vi "x1_move1.vi"() -> (0 "Enum":T1(ring))   [LabVIEW 2016]
uses:
  <vilib>/NXT/Block Support/NXT_OutputPort.ctl
  <vilib>/NXT/NXTIO Xnodes/NXTIONodeSubVIs/NXTMotorRunDistance.vi
  <vilib>/NXT/NXTIO Xnodes/NXTIONodeSubVIs/NXTMoveMotors.vi
  <vilib>/NXT/NXTIO Xnodes/NXTIONodeSubVIs/LEGOMotorStatus.vi
  <vilib>/NXT/NXTIO Xnodes/NXTIONodeSubVIs/NXTStopMotors.vi
  <vilib>/NXT/NXTIO Xnodes/NXTIONodeSubVIs/LEGOResetMotors.vi
  <vilib>/NXT/NXTIO Xnodes/AddressXNode/NXTIOAddress.xnode
  <vilib>/NXT/Subs/LVHSConnector.ctl
  <vilib>/NXT/NXTIO Xnodes/NXTIOXNode/NXTIO.xnode
  <vilib>/NXT/LegoClasses/BrickReference/BrickReference.lvclass
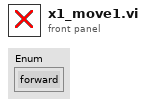
[diagram p1: front panel]
types:
  T1 = enum16{"forward", "mark", "pause", "up", "return", "end"}
  T2 = typedef "NXT_OutputPort.ctl" = u8
  T3 = cluster{"Output Port":T2, "Output Port 2":T2, "Output Port 3":T2}
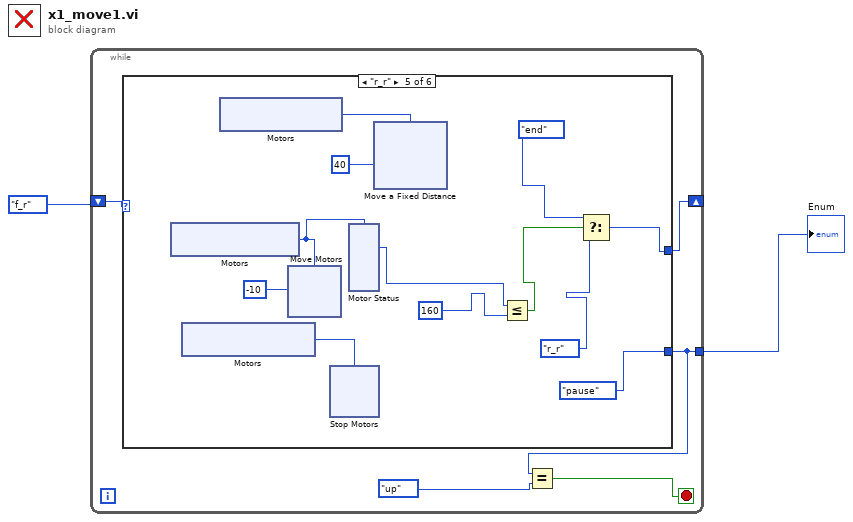
[diagram p0: block diagram]
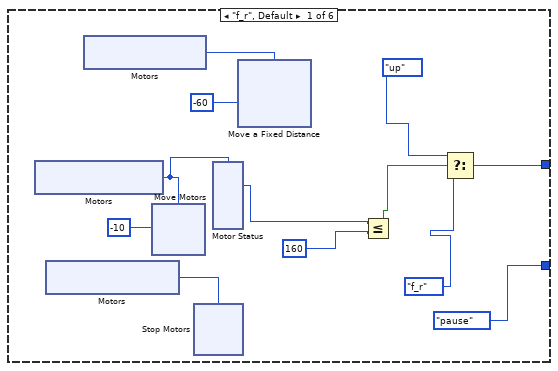
[diagram p2: hidden frame]
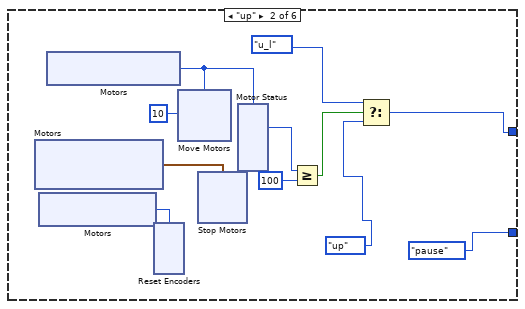
[diagram p3: hidden frame]
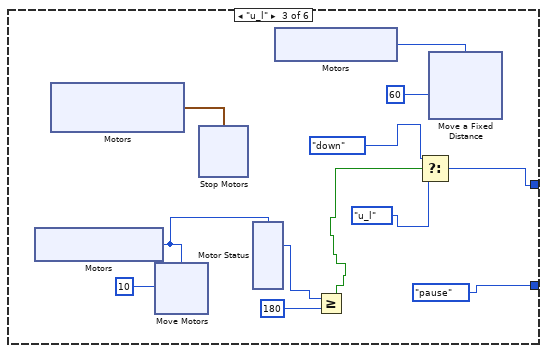
[diagram p4: hidden frame]
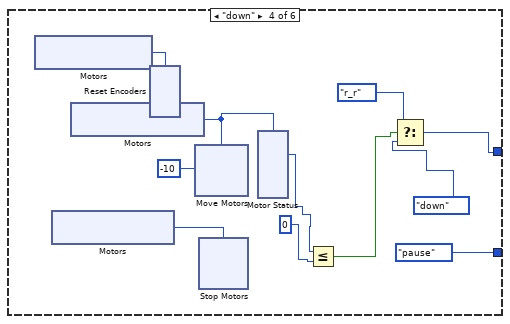
[diagram p5: hidden frame]
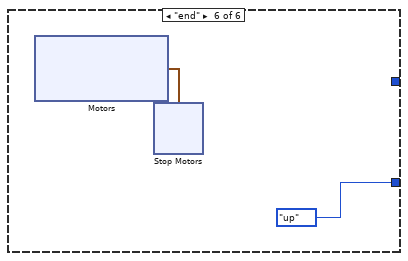
[diagram p6: hidden frame]
diagram:
  n1 = while {
    shift-right: [w6] -> _
    shift-left: enum16{"f_r", "up", "u_l", "down", "r_r", "end"}."f_r" -> [w7]
    tunnel: [w3] -> w1
    stop <- w5 stop-if-true
    n2 = case shown="\"r_r\"" w7 {
      tunnel: [w14 w56 w99 w137 w178 _] -> w6
      tunnel: [T1."pause" T1."pause" T1."pause" T1."pause" T1."pause" T1."up"] -> w3
      frame "f_r", Default {
        n3 = xnode "Motors"() -> ("Motor"=w16:T2)
        n4 = xnode "Motors"() -> ("Motor"=w15:T2)
        n5 = xnode "Motors"() -> ("Motor"=w18:T2)
        n6 = xnode "Move Motors"("Power/Speed 1"=i8 -10, "Motors"=w16) -> ()  [unwired: 1 in, 1 out]
        n7 = xnode "Stop Motors"("Motors"=w15) -> ()  [unwired: 1 in, 1 out]
        n8 = xnode "Motor Status"("Motors"=w16) -> ("Position 1"=w10:i32)  [unwired: 1 in, 2 out]
        n9 = xnode "Move a Fixed Distance"("Speed 1"=i8 -60, "Motors"=w18) -> ()  [unwired: 2 in, 1 out]
        n10 = Less Or Equal?(x=w10, y=160) -> (x <= y?=w11:bool)
        n11 = Select(t=enum16{"f_r", "up", "u_l", "down", "r_r", "end"}."up", s=w11, f=enum16{"f_r", "up", "u_l", "down", "r_r", "end"}."f_r") -> (s? t:f=w14:enum16{"f_r", "up", "u_l", "down", "r_r", "end"})
      }
      frame "up" {
        n12 = xnode "Motors"() -> ("Motor"=w62:cluster{"Port":T2, "Port":T2})
        n13 = xnode "Motors"() -> ("Motor"=w57:T2)
        n14 = xnode "Motors"() -> ("Motor"=w59:T2)
        n15 = xnode "Reset Encoders"("Motors"=w57) -> ()  [unwired: 1 in, 1 out]
        n16 = xnode "Move Motors"("Power/Speed 1"=i8 10, "Motors"=w59) -> ()  [unwired: 1 in, 1 out]
        n17 = xnode "Stop Motors"("Motors"=w62) -> ()  [unwired: 1 in, 1 out]
        n18 = xnode "Motor Status"("Motors"=w59) -> ("Position 1"=w60:i32)  [unwired: 1 in, 2 out]
        n19 = Greater Or Equal?(x=w60, y=100) -> (x >= y?=w61:bool)
        n20 = Select(t=enum16{"f_r", "up", "u_l", "down", "r_r", "end"}."u_l", s=w61, f=enum16{"f_r", "up", "u_l", "down", "r_r", "end"}."up") -> (s? t:f=w56:enum16{"f_r", "up", "u_l", "down", "r_r", "end"})
      }
      frame "u_l" {
        n21 = xnode "Motors"() -> ("Motor"=w101:T2)
        n22 = xnode "Motors"() -> ("Motor"=w100:cluster{"Port":T2, "Port":T2})
        n23 = xnode "Move Motors"("Power/Speed 1"=i8 10, "Motors"=w101) -> ()  [unwired: 1 in, 1 out]
        n24 = xnode "Stop Motors"("Motors"=w100) -> ()  [unwired: 1 in, 1 out]
        n25 = xnode "Motor Status"("Motors"=w101) -> ("Position 1"=w92:i32)  [unwired: 1 in, 2 out]
        n26 = xnode "Motors"() -> ("Motor"=w94:T2)
        n27 = Greater Or Equal?(x=w92, y=180) -> (x >= y?=w93:bool)
        n28 = Select(t=enum16{"f_r", "up", "u_l", "down", "r_r", "end"}."down", s=w93, f=enum16{"f_r", "up", "u_l", "down", "r_r", "end"}."u_l") -> (s? t:f=w99:enum16{"f_r", "up", "u_l", "down", "r_r", "end"})
        n29 = xnode "Move a Fixed Distance"("Speed 1"=i8 60, "Motors"=w94) -> ()  [unwired: 2 in, 1 out]
      }
      frame "down" {
        n30 = xnode "Motors"() -> ("Motor"=w142:T2)
        n31 = xnode "Motors"() -> ("Motor"=w146:T2)
        n32 = xnode "Motors"() -> ("Motor"=w144:T2)
        n33 = xnode "Reset Encoders"("Motors"=w142) -> ()  [unwired: 1 in, 1 out]
        n34 = xnode "Move Motors"("Power/Speed 1"=i8 -10, "Motors"=w144) -> ()  [unwired: 1 in, 1 out]
        n35 = xnode "Stop Motors"("Motors"=w146) -> ()  [unwired: 1 in, 1 out]
        n36 = xnode "Motor Status"("Motors"=w144) -> ("Position 1"=w143:i32)  [unwired: 1 in, 2 out]
        n37 = Less Or Equal?(x=w143, y=0) -> (x <= y?=w140:bool)
        n38 = Select(t=enum16{"f_r", "up", "u_l", "down", "r_r", "end"}."r_r", s=w140, f=enum16{"f_r", "up", "u_l", "down", "r_r", "end"}."down") -> (s? t:f=w137:enum16{"f_r", "up", "u_l", "down", "r_r", "end"})
      }
      frame "r_r" {
        n39 = xnode "Motors"() -> ("Motor"=w182:T2)
        n40 = xnode "Motors"() -> ("Motor"=w181:T2)
        n41 = xnode "Motors"() -> ("Motor"=w184:T2)
        n42 = xnode "Move Motors"("Power/Speed 1"=i8 -10, "Motors"=w182) -> ()  [unwired: 1 in, 1 out]
        n43 = xnode "Stop Motors"("Motors"=w181) -> ()  [unwired: 1 in, 1 out]
        n44 = xnode "Motor Status"("Motors"=w182) -> ("Position 1"=w176:i32)  [unwired: 1 in, 2 out]
        n45 = xnode "Move a Fixed Distance"("Speed 1"=i8 40, "Motors"=w184) -> ()  [unwired: 2 in, 1 out]
        n46 = Less Or Equal?(x=w176, y=160) -> (x <= y?=w174:bool)
        n47 = Select(t=enum16{"f_r", "up", "u_l", "down", "r_r", "end"}."end", s=w174, f=enum16{"f_r", "up", "u_l", "down", "r_r", "end"}."r_r") -> (s? t:f=w178:enum16{"f_r", "up", "u_l", "down", "r_r", "end"})
      }
      frame "end" {
        n48 = xnode "Motors"() -> ("Motor"=w220:cluster{"Port":T2, "Port":T2, "Port":T2})
        n49 = xnode "Stop Motors"("Motors"=w220) -> ()  [unwired: 1 in, 1 out]
      }
    }
    n50 = Equal?(x=w3, y=T1."up") -> (x = y?=w5:bool)
  }
  "Enum" <- w1
